vi "GUI_HTU_Steering_Magnets.vi"() -> ()   [LabVIEW 2020]
uses:
  Shared/GUI_Template/GUI_master/tcp_new_data_event.ctl
  Shared/GUI_Template/GUI_master/tcp new data cluster.ctl
panel:
  in  "GUIdevice 18":string="U_VS5V"
  in  "GUIdevice 17":string="U_VS5H"
  in  "Voltage::17":dbl caption="VS5H Voltage" min=-10.0 max=10.0
  in  "Voltage::18":dbl caption="VS5V Voltage" min=-10.0 max=10.0
  in  "Enable_Output::18":enum16{"on", "off"}(ring) caption="Enable VS5V"
  in  "Enable_Output::17":enum16{"on", "off"}(ring) caption="Enable VS5H"
  in  "Current::17":dbl caption="VS5H Current" min=-5.0 max=5.0
  in  "Current::18":dbl caption="VS5V Current" min=-5.0 max=5.0
  in  "Voltage::15":dbl caption="VS4H Voltage" min=-10.0 max=10.0
  in  "Voltage::16":dbl caption="VS4V Voltage" min=-10.0 max=10.0
  in  "Enable_Output::16":enum16{"on", "off"}(ring) caption="Enable VS4V"
  in  "Enable_Output::15":enum16{"on", "off"}(ring) caption="Enable VS4H"
  in  "Current::15":dbl caption="VS4H Current" min=-5.0 max=5.0
  in  "Current::16":dbl caption="VS4V Current" min=-5.0 max=5.0
  in  "Voltage::13":dbl caption="VS3H Voltage" min=-10.0 max=10.0
  in  "Voltage::14":dbl caption="VS3V Voltage" min=-10.0 max=10.0
  in  "Enable_Output::14":enum16{"on", "off"}(ring) caption="Enable VS3V"
  in  "Enable_Output::13":enum16{"on", "off"}(ring) caption="Enable VS3H"
  in  "Current::13":dbl caption="VS3H Current" min=-5.0 max=5.0
  in  "Current::14":dbl caption="VS3V Current" min=-5.0 max=5.0
  in  "Voltage::11":dbl caption="VS2H Voltage" min=-10.0 max=10.0
  in  "Voltage::12":dbl caption="VS2V Voltage" min=-10.0 max=10.0
  in  "Enable_Output::12":enum16{"on", "off"}(ring) caption="Enable VS2V"
  in  "Enable_Output::11":enum16{"on", "off"}(ring) caption="Enable VS2H"
  in  "Current::11":dbl caption="VS2H Current" min=-5.0 max=5.0
  in  "Current::12":dbl caption="VS2V Current" min=-5.0 max=5.0
  in  "GUIdevice 16":string="U_VS4V"
  in  "GUIdevice 15":string="U_VS4H"
  in  "GUIdevice 14":string="U_VS3V"
  in  "GUIdevice 13":string="U_VS3H"
  in  "GUIdevice 12":string="U_VS2V"
  in  "GUIdevice 11":string="U_VS2H"
  in  "GUIdevice 10":string="U_VS1V"
  in  "GUIdevice 9":string="U_VS1H"
  in  "Voltage::9":dbl caption="VS1H Voltage" min=-10.0 max=10.0
  in  "Voltage::10":dbl caption="VS1V Voltage" min=-10.0 max=10.0
  in  "Enable_Output::10":enum16{"on", "off"}(ring) caption="Enable VS1V"
  in  "Enable_Output::9":enum16{"on", "off"}(ring) caption="Enable VS1H"
  in  "Current::9":dbl caption="VS1H Current" min=-5.0 max=5.0
  in  "Current::10":dbl caption="VS1V Current" min=-5.0 max=5.0
  in  "GUIdevice 8":string="U_S4V"
  in  "GUIdevice 7":string="U_S4H"
  in  "Voltage::7":dbl caption="S4H Voltage" min=-10.0 max=10.0
  in  "Voltage::8":dbl caption="S4V Voltage" min=-10.0 max=10.0
  in  "Enable_Output::8":enum16{"on", "off"}(ring) caption="Enable S4V"
  in  "Enable_Output::7":enum16{"on", "off"}(ring) caption="Enable S4H"
  in  "Current::7":dbl caption="S4H Current" min=-5.0 max=5.0
  in  "Current::8":dbl caption="S4V Current" min=-5.0 max=5.0
  in  "GUIdevice 6":string="U_S3V"
  in  "GUIdevice 5":string="U_S3H"
  in  "Voltage::5":dbl caption="S3H Voltage" min=-10.0 max=10.0
  in  "Voltage::6":dbl caption="S3V Voltage" min=-10.0 max=10.0
  in  "Enable_Output::6":enum16{"on", "off"}(ring) caption="Enable S3V"
  in  "Enable_Output::5":enum16{"on", "off"}(ring) caption="Enable S3H"
  in  "Current::5":dbl caption="S3H Current" min=-5.0 max=5.0
  in  "Current::6":dbl caption="S3V Current" min=-5.0 max=5.0
  in  "Voltage::3":dbl caption="S2H Voltage" min=-10.0 max=10.0
  in  "Voltage::4":dbl caption="S2V Voltage" min=-10.0 max=10.0
  in  "Enable_Output::4":enum16{"on", "off"}(ring) caption="Enable S2V"
  in  "Enable_Output::3":enum16{"on", "off"}(ring) caption="Enable S2H"
  in  "Current::3":dbl caption="S2H Current" min=-5.0 max=5.0
  in  "Current::4":dbl caption="S2V Current" min=-5.0 max=5.0
  in  "GUIdevice 4":string="U_S2V"
  in  "GUIdevice 3":string="U_S2H"
  in  "Voltage::1":dbl caption="S1H Voltage" min=-10.0 max=10.0
  in  "Voltage::2":dbl caption="S1V Voltage" min=-10.0 max=10.0
  in  "Enable_Output::2":enum16{"on", "off"}(ring) caption="Enable S1V"
  in  "Enable_Output::1":enum16{"on", "off"}(ring) caption="Enable S1H"
  in  "Current::1":dbl caption="S1H Current" min=-5.0 max=5.0
  in  "Current::2":dbl caption="S1V Current" min=-5.0 max=5.0
  out "error IO 2":errorcluster
  out "tcp data event":T1
  in  "UDP error message":string
  in  "GUIdevice 2":string="U_S1V"
  in  "GUIdevice 1":string="U_S1H"
  in  "stop":bool
  # "Energy"
  # "HTU Steering Magnets"
  # "S1H"
  # "S1V"
  # "S2H"
  # "S2V"
  # "S3H"
  # "S3V"
  # "S4H"
  # "S4V"
  # "Enable output"
  # "Current"
  # "Voltage"
  # "VS1H"
  # "VS1V"
  # "VS2H"
  # "VS2V"
  # "VS3H"
  # "VS3V"
  # "VS4H"
  # "VS4V"
  # "VS5H"
  # "VS5V"
  # "Enable output"
  # "Current"
  # "Voltage"
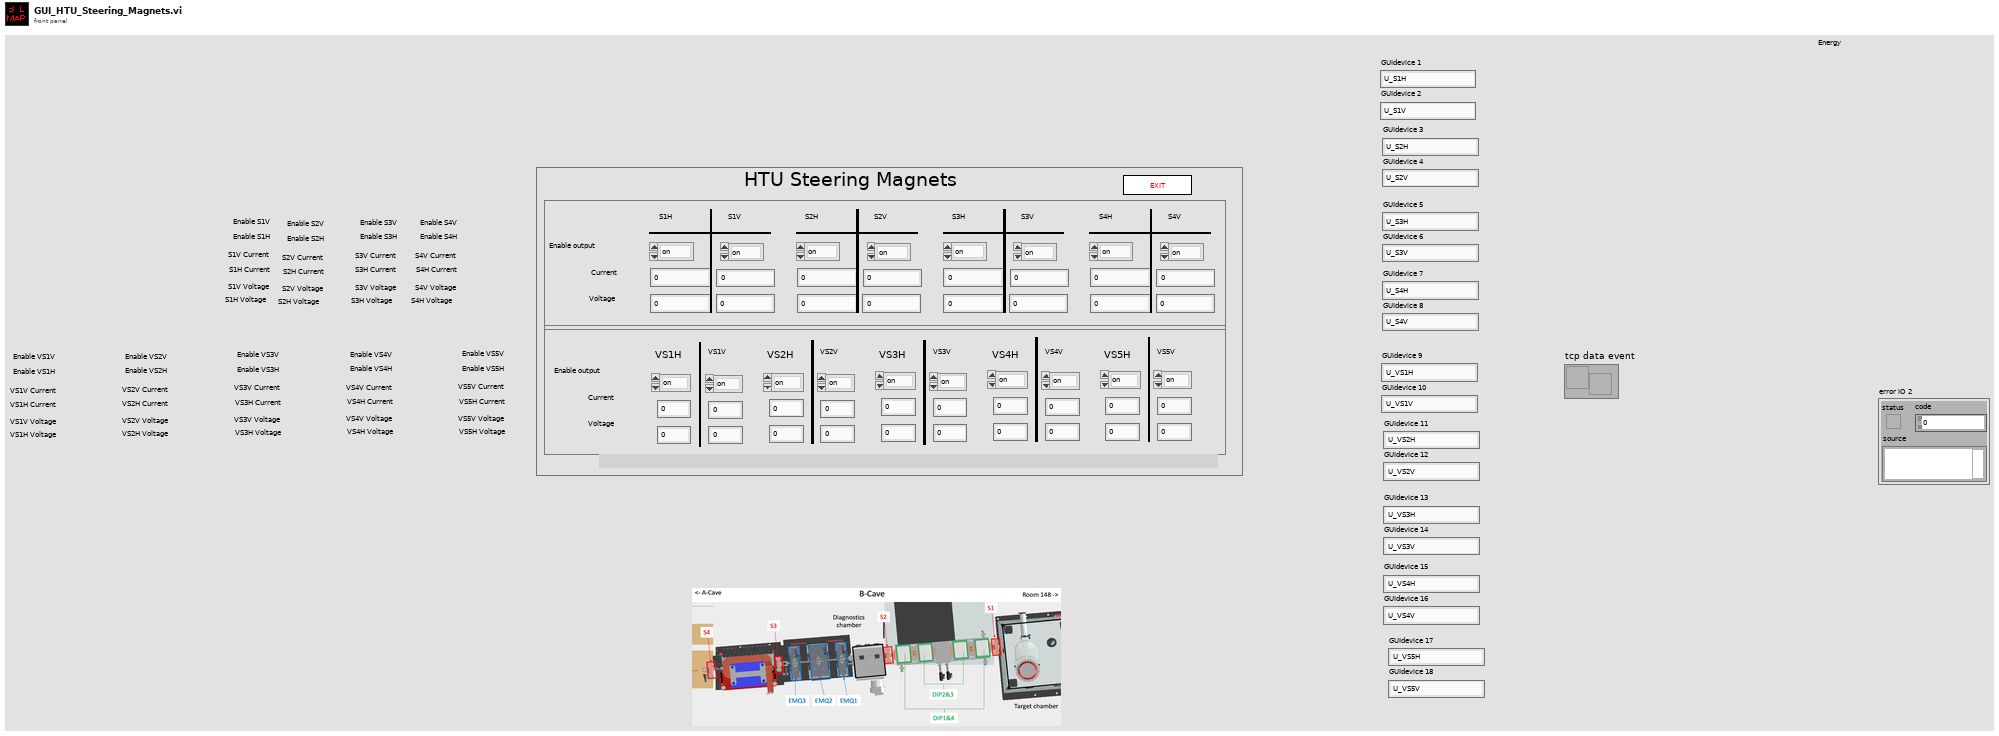
[diagram p1: front panel]
types:
  T1 = typedef "tcp_new_data_event.ctl" = refnum<user-event>
  T2 = typedef "tcp new data cluster.ctl" = cluster{"EventEnum":enum16{"new data", "connection status update"}, "Device name":string}
  T3 = enum32{"invalid app kind", "Development System", "Run Time System", "Student Edition", "Embedded LabVIEW", "Evaluation", "Custom"}
  T4 = enum32{"Invalid", "Standard", "Closed", "Hidden", "Minimized", "Maximized"}
  T5 = cluster{"Core":cluster{"Current VI Reference":refnum<vi>, "Close Panel on Exit?":bool}}
  T6 = cluster{"Current VI Reference":refnum<vi>, "Close Panel on Exit?":bool}
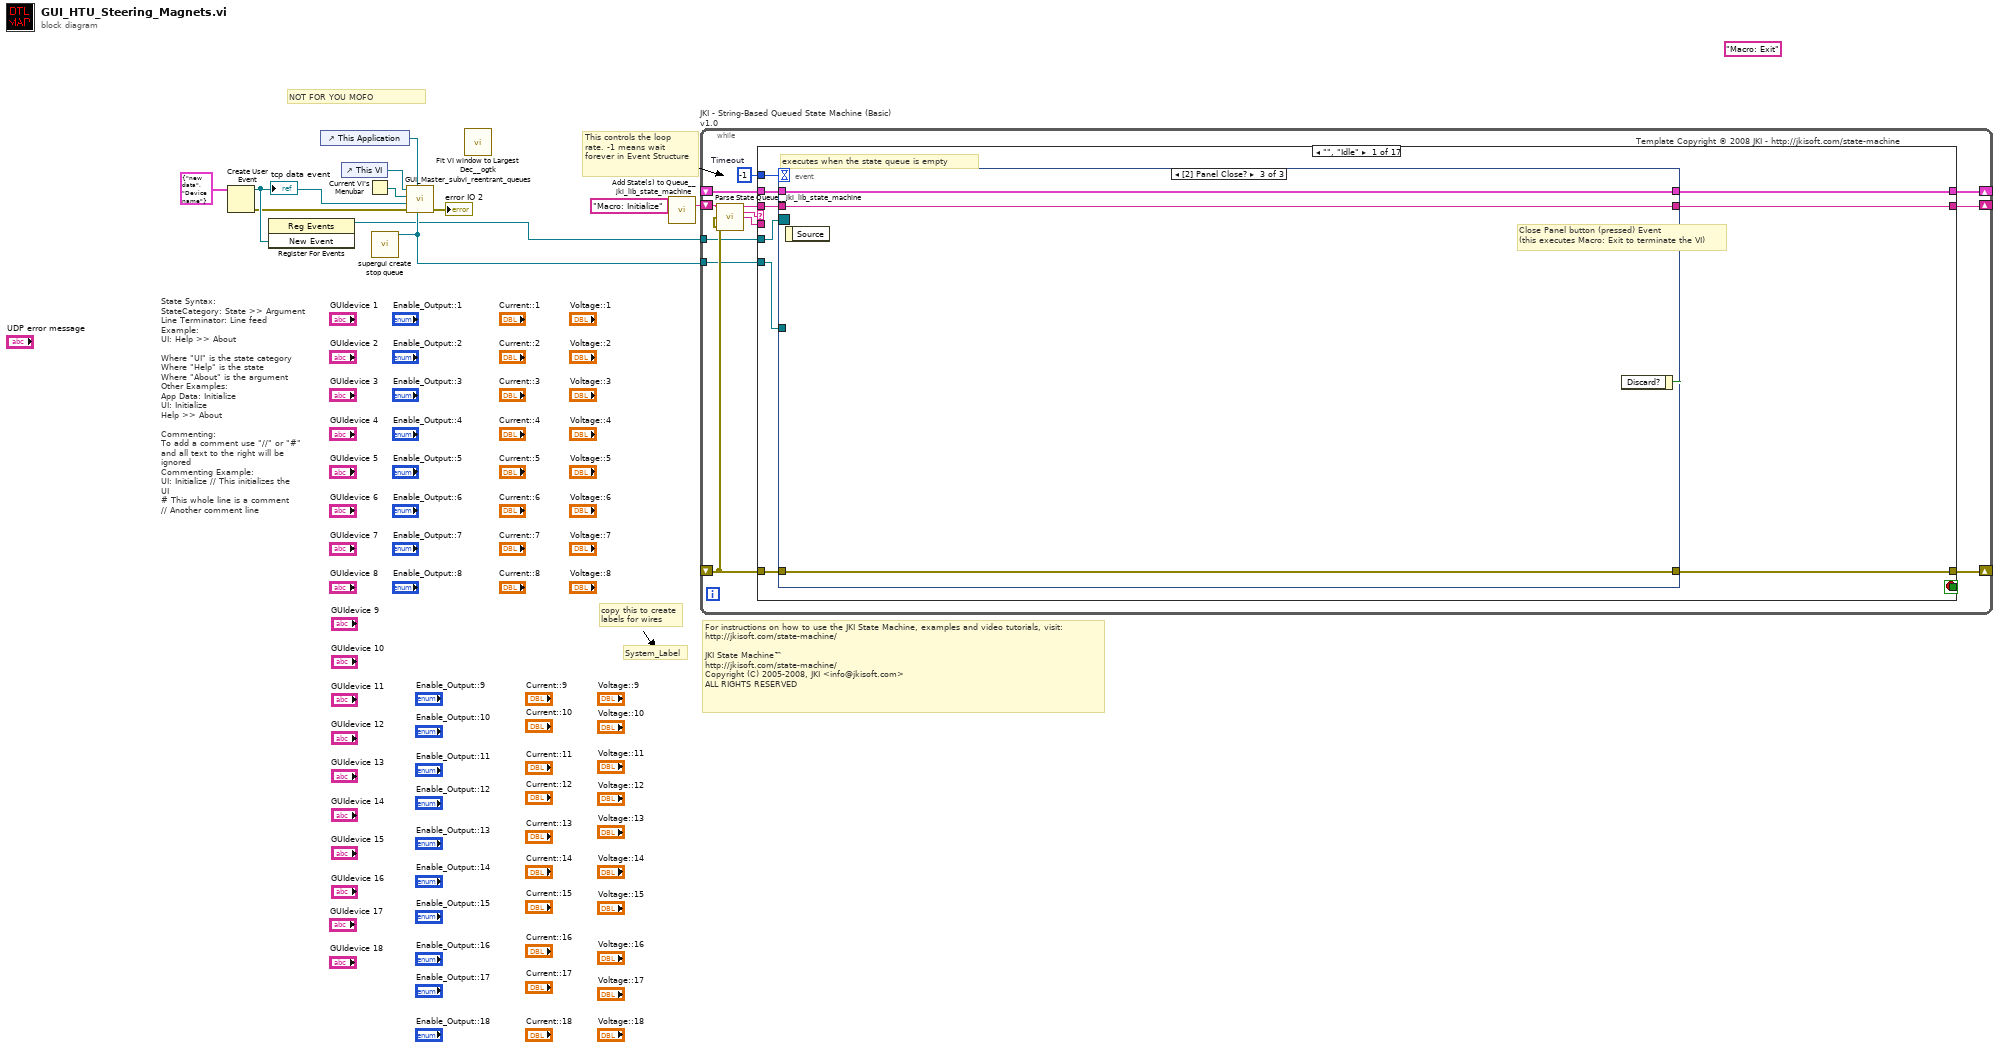
[diagram p0: block diagram]
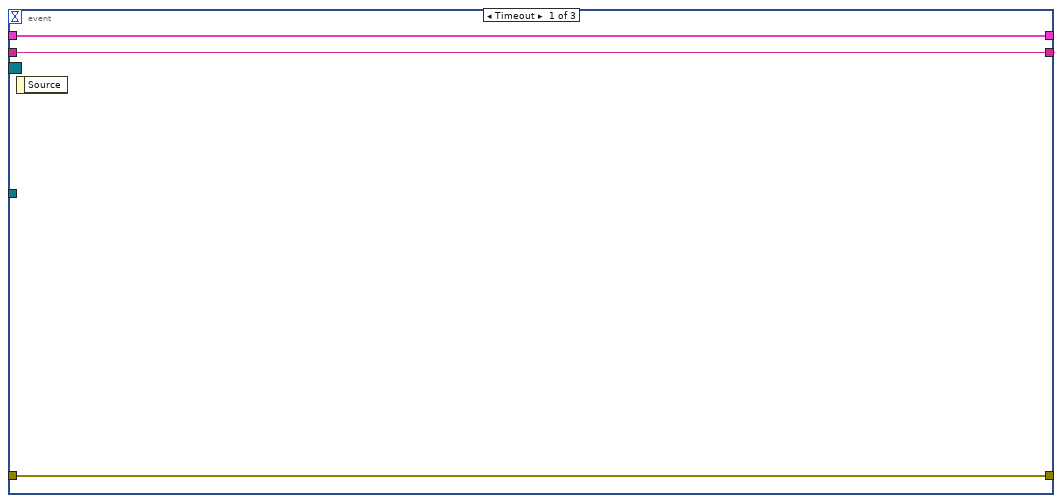
[diagram p2: hidden frame]
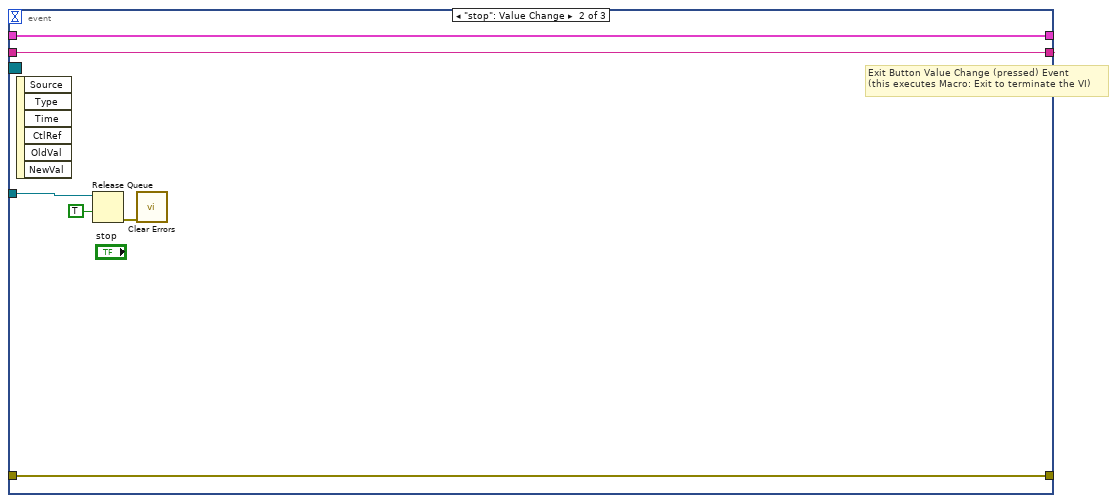
[diagram p3: hidden frame]
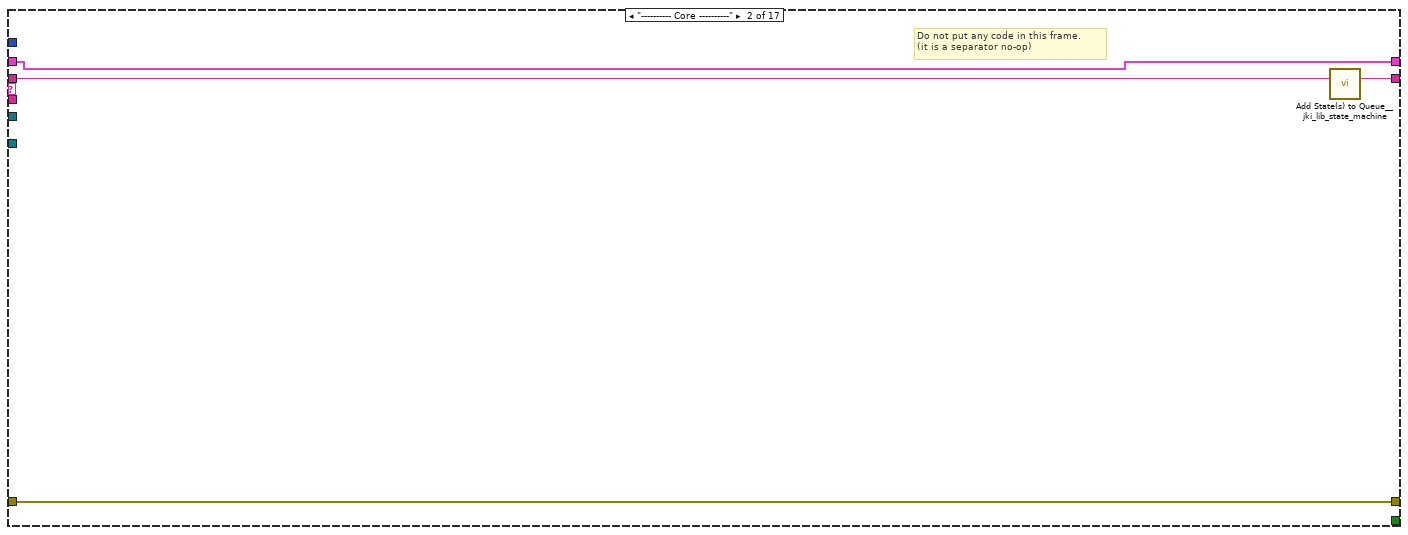
[diagram p4: hidden frame]
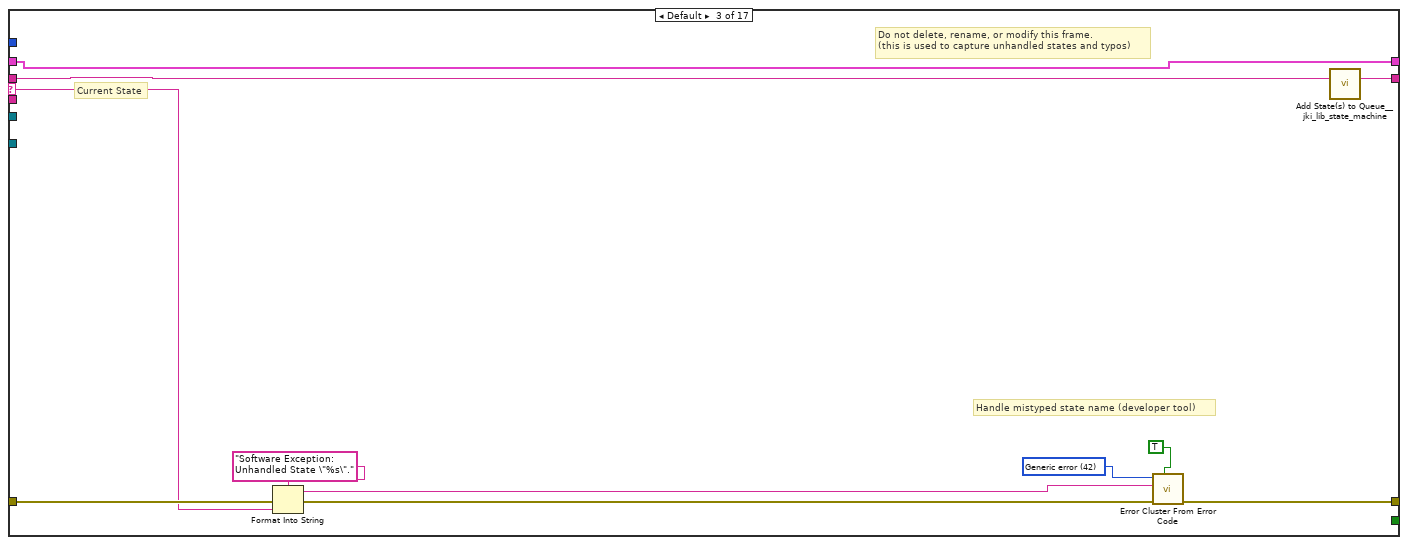
[diagram p5: hidden frame]
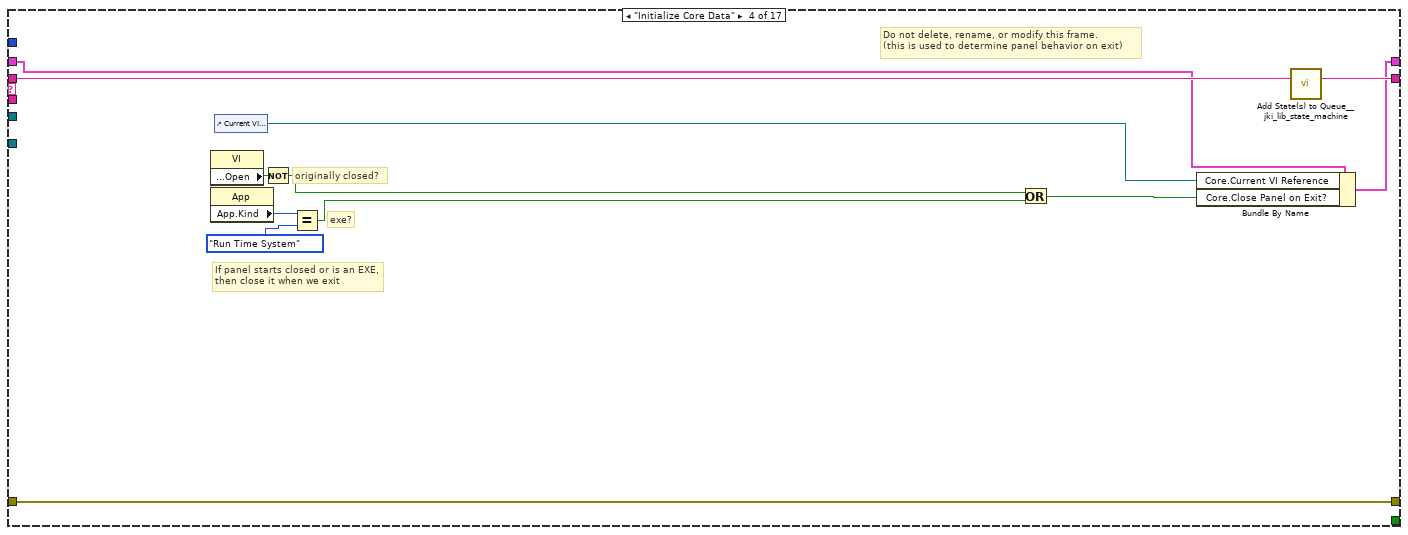
[diagram p6: hidden frame]
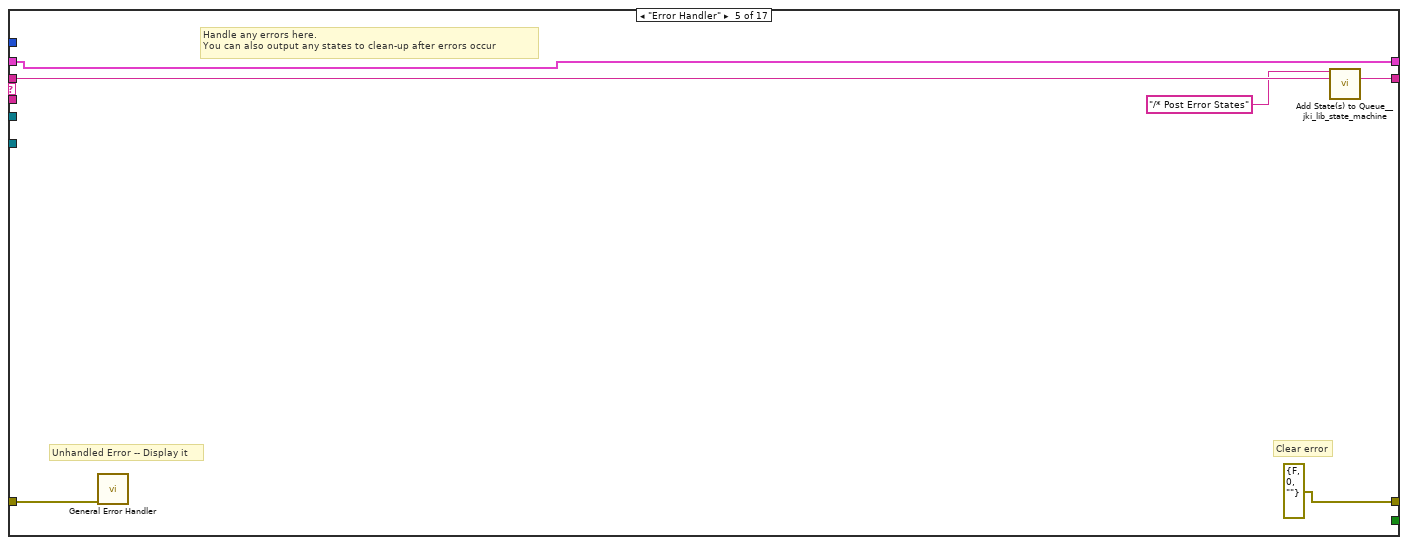
[diagram p7: hidden frame]
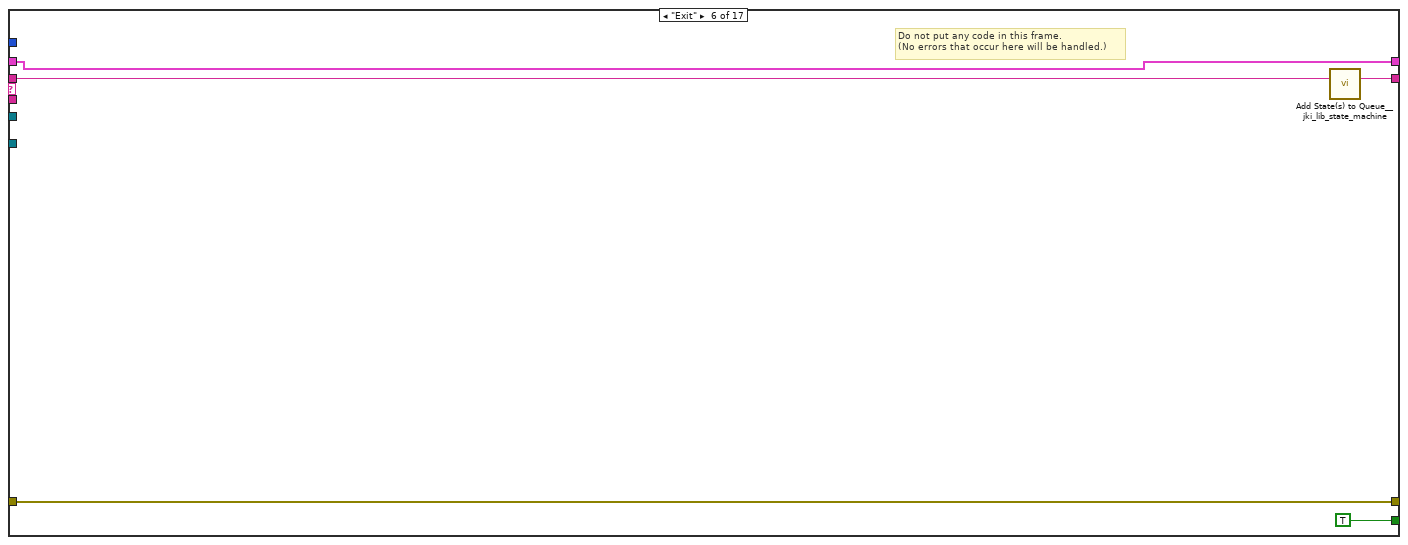
[diagram p8: hidden frame]
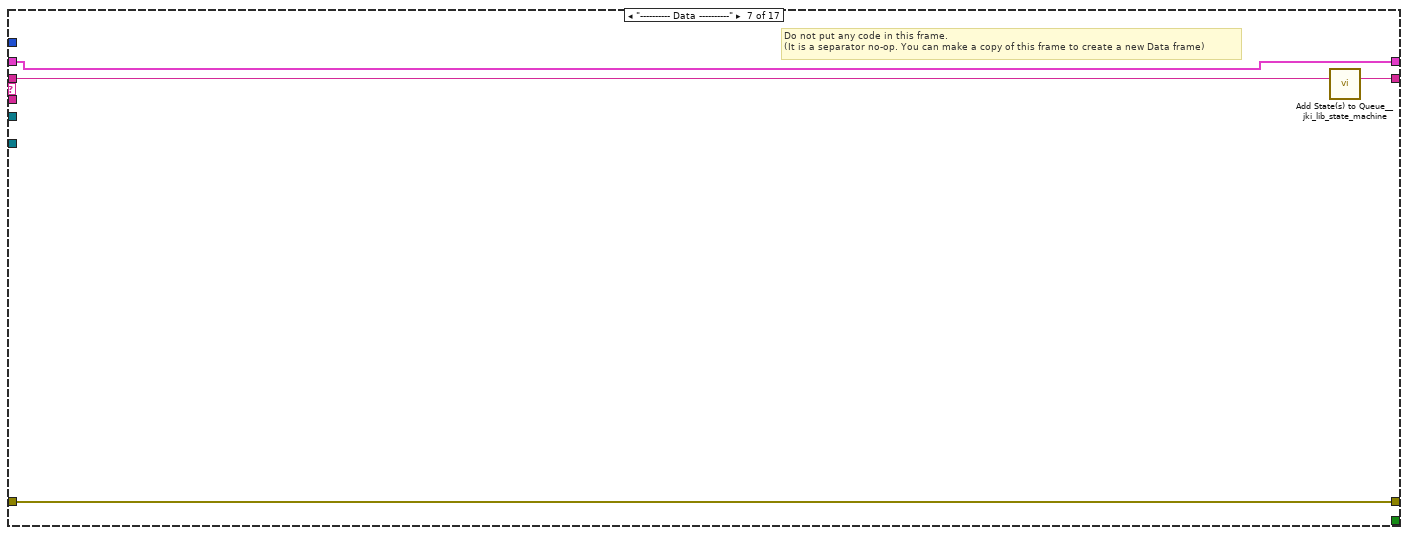
[diagram p9: hidden frame]
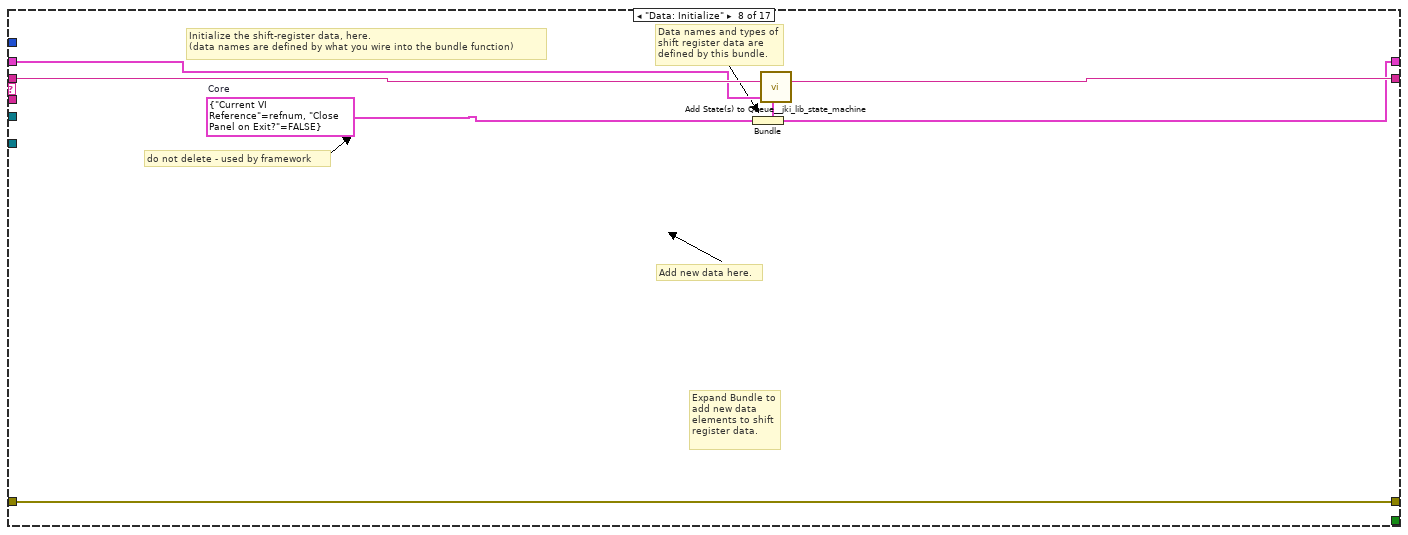
[diagram p10: hidden frame]
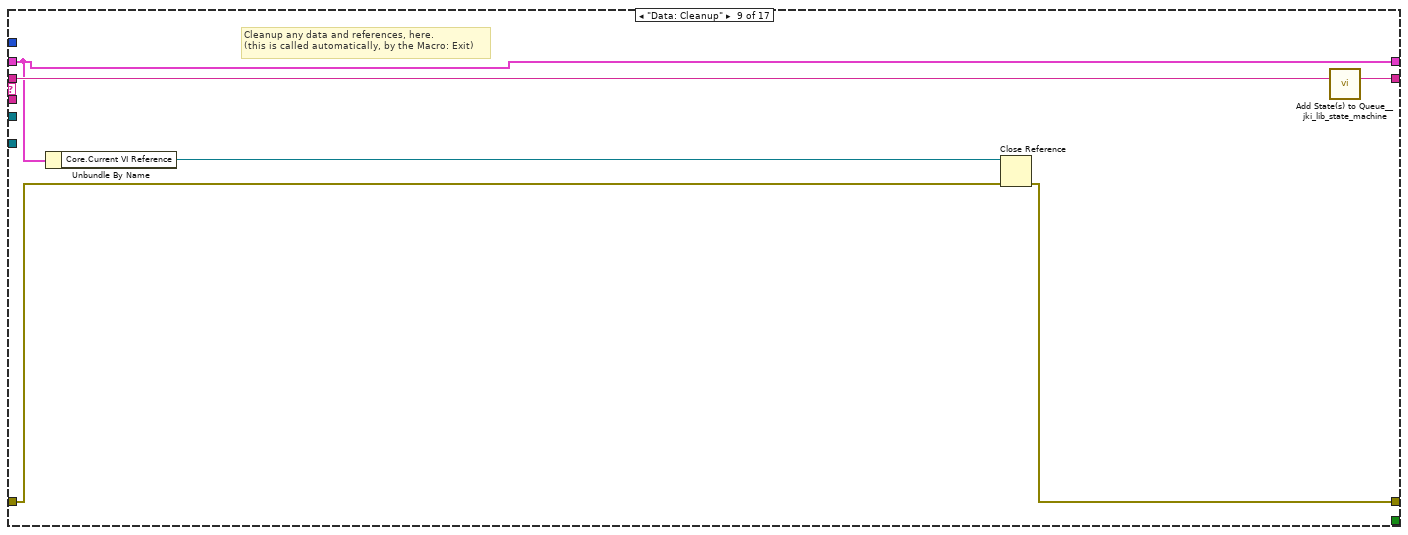
[diagram p11: hidden frame]
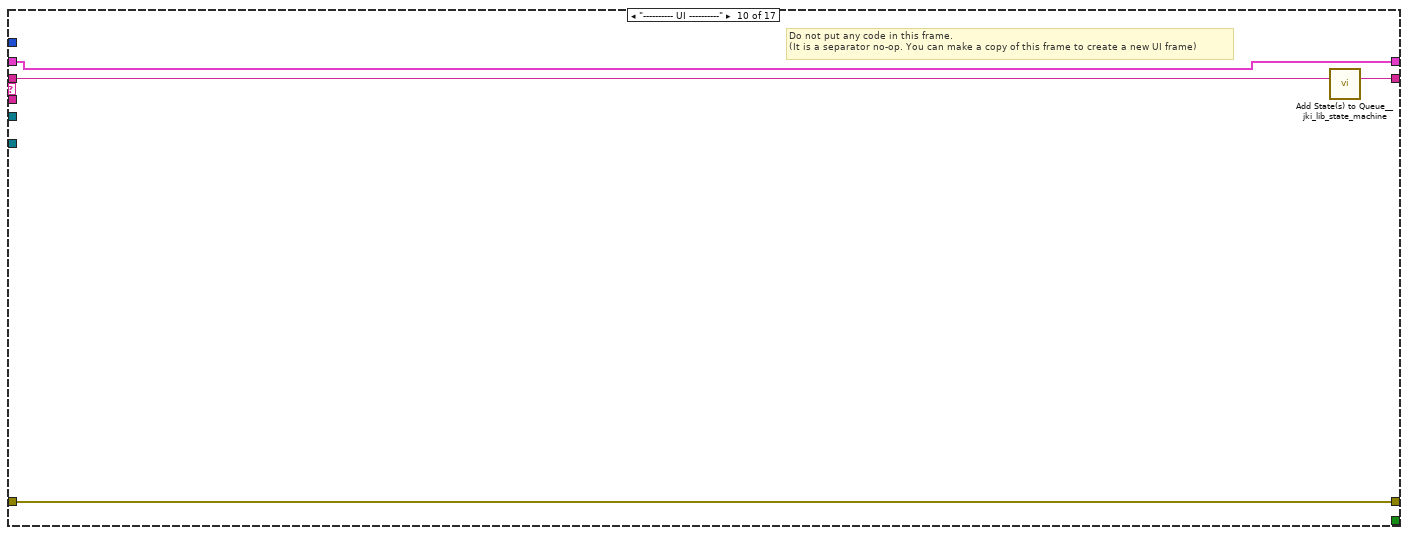
[diagram p12: hidden frame]
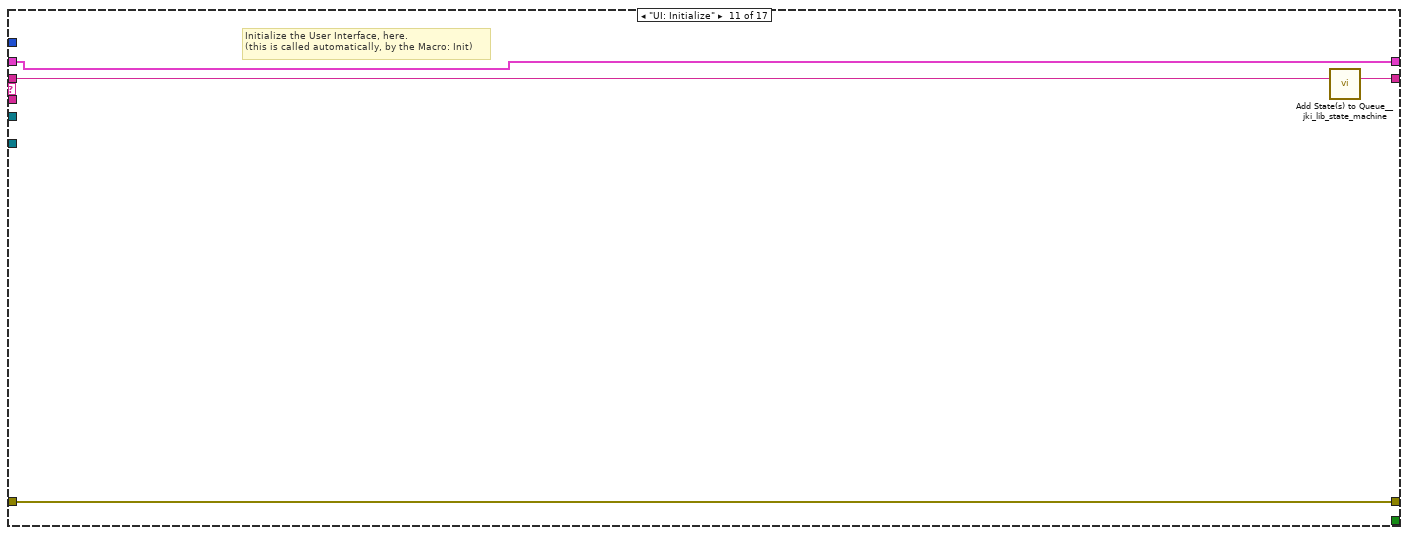
[diagram p13: hidden frame]
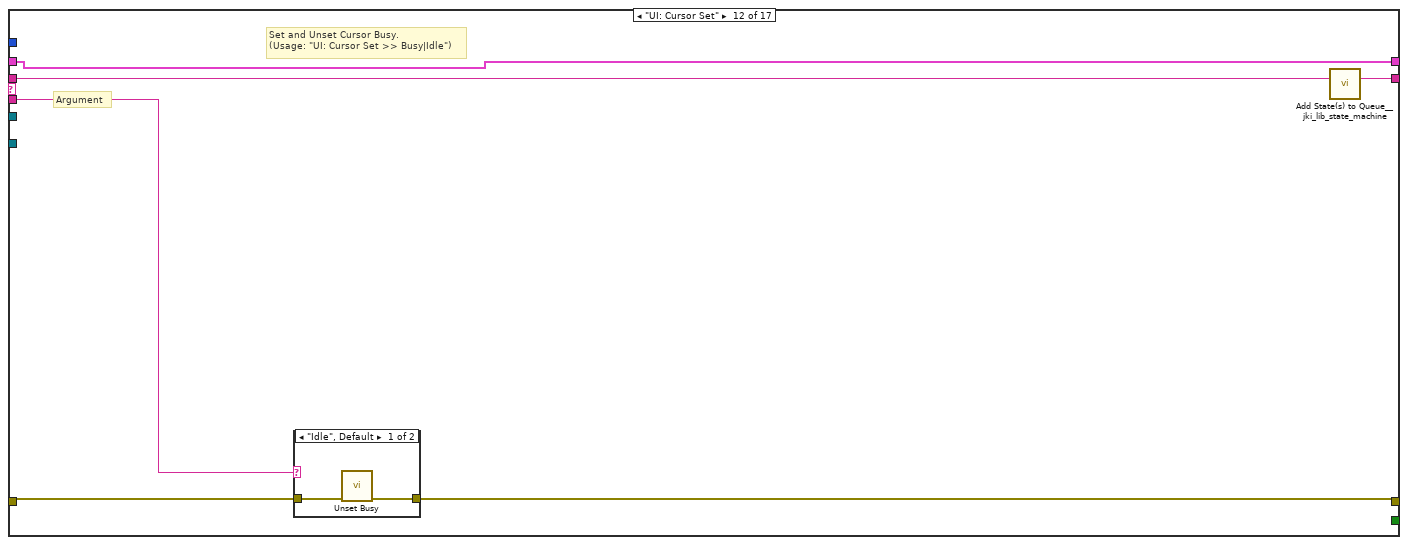
[diagram p14: hidden frame]
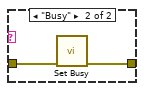
[diagram p15: hidden frame]
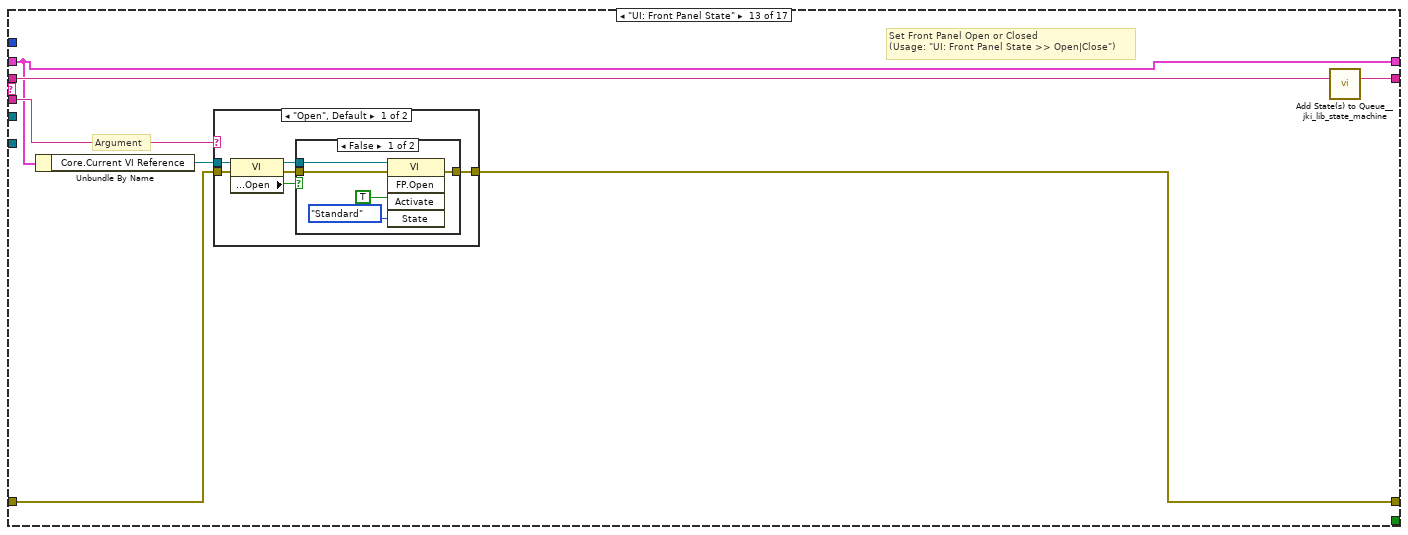
[diagram p16: hidden frame]
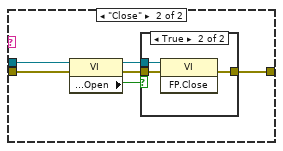
[diagram p18: hidden frame]
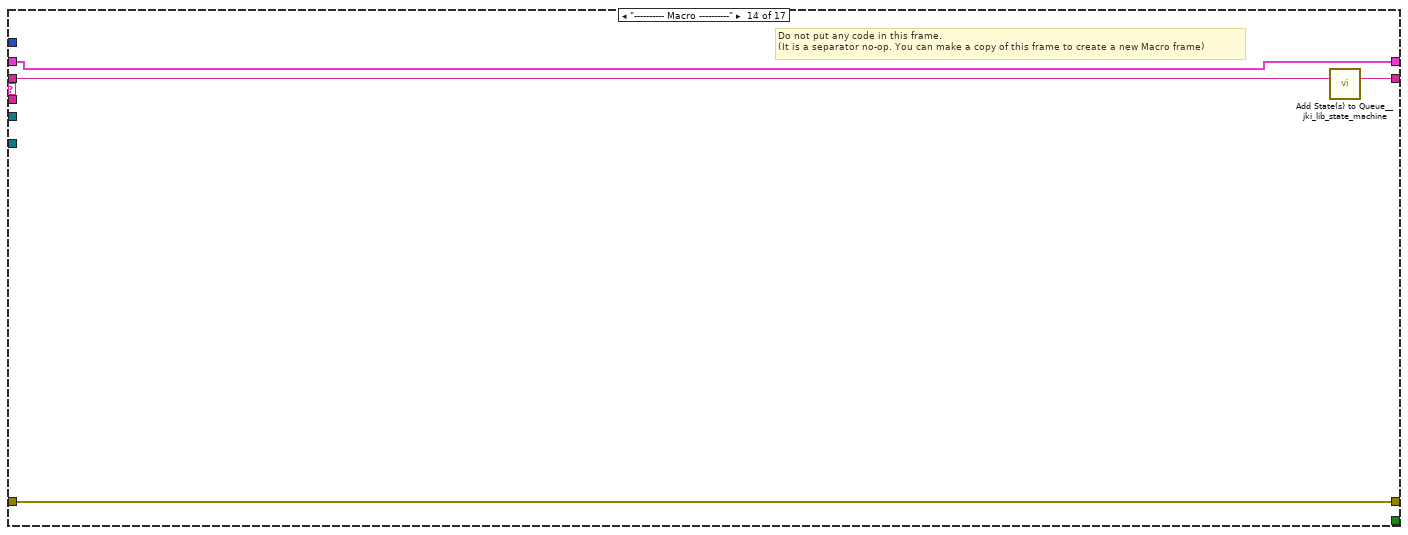
[diagram p20: hidden frame]
diagram:
  (unwired) "Macro: Exit"
  # "For instructions on how to use the JKI State Machine, examples and video tutorials, visit:\nhttp://jkisoft.com/state-machine/\n\nJKI State Machine™\nhttp://jkisoft.com/state-machine/\nCopyright (C) 2005-2008, JKI <info@jkisoft.com>\nALL RIGHTS RESERVED"
  # "State Syntax:\nStateCategory: State >> Argument\nLine Terminator: Line feed\nExample:\nUI: Help >> About\n\nWhere \"UI\" is the state category\nWhere \"Help\" is the state\nWhere \"About\" is the argument\nOther Examples:\nApp Data: Initialize\nUI: Initialize\nHelp >> About\n\nCommenting:\nTo add a comment use \"//\" or \"#\" and all text to the right will be ignored\nCommenting Example:\nUI: Initialize // This initializes the UI\n# This whole line is a comment\n// Another comment line"
  # "copy this to create labels for wires"
  # "This controls the loop rate. -1 means wait forever in Event Structure"
  # "System_Label"
  # "NOT FOR YOU MOFO"
  n1 = Create User Event(user event datatype=T2 {"EventEnum"=enum."new data", "Device name"="Device name"} ("New Event")) -> (user event=w10:refnum<user-event>, error out=w9:errorcluster)  [unwired: 1 in]
  "tcp data event" <- w10
  n2 = register-events(w10) -> (reference out=w1:refnum<event-registration>)  [unwired: 2 in, 1 out]
  n3 = control-ref of="This Application"() -> (w11:refnum<vi>)
  n4 = control-ref of="This VI"() -> (w5:refnum<vi>)
  n5 = Current VI's Menubar() -> (w7:refnum<k9>)
  n6 = call "supergui create stop queue.vi"() -> ("STOP Queue out"=w2:refnum<queue>)  [unwired: 11 in]
  n7 = call "GUI_Master_subvi_reentrant_queues.vi"("STOP Queue in"=w2, "This Application"=w11, "error in (no error)"=w9, "tcp data event"=w10, "Caller menu reference"=w7, "Caller VI ref"=w5) -> ("error out"=→"error IO 2":errorcluster)  [unwired: 5 in]
  n8 = call <userlib>:"Fit VI window to Largest Dec__ogtk.vi"() -> ()  [unwired: 6 in, 2 out]
  n9 = call <vilib>:"Add State(s) to Queue__jki_lib_state_machine.vi"("State(s) in (\"\")"="Macro: Initialize") -> ("States Out"=w3:string)  [unwired: 14 in]
  n10 = while "JKI - String-Based Queued State Machine (Basic) v1.0" {
    shift-right: [w17] -> _
    shift-left: _ -> [w16]
    shift-right: [w20] -> _
    shift-left: _ -> [w14]
    shift-right: [w19] -> _
    shift-left: w3 -> [w21]
    tunnel: w1 -> [w13]
    tunnel: w2 -> [w12]
    stop <- w18 stop-if-true
    w15 = -1  # Timeout
    # "Template Copyright © 2008 JKI - http://jkisoft.com/state-machine"
    n11 = call <vilib>:"Parse State Queue__jki_lib_state_machine.vi"("State Queue"=w21, "Error In (no error)"=w14) -> ("Remaining States"=w23:string, "Current State"=w24:string, "Arguments"=w22:string)  [unwired: 11 in]
    n12 = case shown="\"\", \"Idle\"" w24 {
      selector: w24 -> [_ _ w56 _ _ _ _ _ _ _ _ _ _ _ _ _ _]
      tunnel: w23 -> [w33 w55 w60 w78 w84 w89 w93 w99 w105 w109 w113 w119 w130 w156 w161 w171 w175]
      tunnel: w22 -> [_ _ _ _ _ _ _ _ _ _ _ w114 w125 _ _ _ _]
      tunnel: w16 -> [w31 w52 w58 w68 w81 w87 w90 w95 w100 w106 w111 w117 w124 w153 w158 w162 w172]
      tunnel: [w30 w53 w62 w76 errorcluster {"status"=FALSE, "code"=0, "source"=""} ("error out") w86 w91 w97 w102 w107 w110 w115 w127 w154 w159 w169 w173] -> w20
      tunnel: w14 -> [w29 w53 w61 w76 w80 w86 w91 w97 w103 w107 w110 w116 w128 w154 w159 w169 w173]
      tunnel: [w32 w54 w59 w77 w83 w88 w92 w98 w104 w108 w112 w118 w129 w155 w160 w170 w174] -> w19
      tunnel: [_ _ _ _ _ TRUE _ _ _ _ _ _ _ _ _ _ _] -> w18
      tunnel: [w25 w52 w58 w67 w81 w87 w90 w94 w100 w106 w111 w117 w124 w153 w158 w162 w172] -> w17
      tunnel: w15 -> [w28 _ _ _ _ _ _ _ _ _ _ _ _ _ _ _ _]
      tunnel: w13 -> [w27 _ _ _ _ _ _ _ _ _ _ _ _ _ _ _ _]
      tunnel: w12 -> [w26 _ _ _ _ _ _ _ _ _ _ _ _ _ _ _ _]
      frame "", "Idle" {
        # "executes when the state queue is empty"
        n13 = event shown="[2] Panel Close?" {
          selector: w27 -> [_ _ _]
          dyn-events: _ -> [_ _ _]
          timeout: w28 -> [_ _ _]
          tunnel: w33 -> [w37 w45 w51]
          tunnel: [w36 w44 w50] -> w32
          tunnel: w31 -> [w34 w42 w48]
          tunnel: [w35 w43 w49] -> w30
          tunnel: w29 -> [w35 w43 w49]
          tunnel: [w34 w42 w48] -> w25
          tunnel: w26 -> [_ w39 _]
          event Timeout {
            n14 = event-data() -> ()  [unwired: 1 in, 1 out]
            n15 = call <vilib>:"Add State(s) to Queue__jki_lib_state_machine.vi"("State(s) in (\"\")"=w37) -> ("States Out"=w36:string)  [unwired: 14 in]
          }
          event "stop": Value Change {
            # "Exit Button Value Change (pressed) Event\n(this executes Macro: Exit to terminate the VI)"
            n16 = event-data() -> ()  [unwired: 1 in, 6 out]
            n17 = Release Queue(queue=w39, force destroy? (F)=TRUE) -> (error out=w40:errorcluster)  [unwired: 1 in, 2 out]
            n18 = call <vilib>:"Clear Errors.vi"("error in (no error)"=w40) -> ()  [unwired: 5 in, 2 out]
            n19 = call <vilib>:"Add State(s) to Queue__jki_lib_state_machine.vi"("State(s) in Front (\"\")"="Macro: Exit", "State(s) in (\"\")"=w45) -> ("States Out"=w44:string)  [unwired: 13 in]
          }
          event Panel Close? {
            # "Discard the event because we'll close the front panel ourselves in Macro: Exit"
            # "Close Panel button (pressed) Event\n(this executes Macro: Exit to terminate the VI)"
            n20 = event-data() -> ()  [unwired: 1 in, 1 out]
            n21 = event-data("Discard?"=TRUE) -> ()  [unwired: 1 in, 1 out]
            n22 = call <vilib>:"Add State(s) to Queue__jki_lib_state_machine.vi"("State(s) in Front (\"\")"="Macro: Exit", "State(s) in (\"\")"=w51) -> ("States Out"=w50:string)  [unwired: 13 in]
          }
        }
      }
      frame "---------- Core ----------" {
        # "Do not put any code in this frame.\n(it is a separator no-op)"
        n23 = call <vilib>:"Add State(s) to Queue__jki_lib_state_machine.vi"("State(s) in (\"\")"=w55) -> ("States Out"=w54:string)  [unwired: 14 in]
      }
      frame Default {
        w65 = 42 items=["No error", "Argument error", "Memory is full", "Out of zone", "End of file", "File already open", "Generic file I/O error", "File not found", "File permission error", "Disk is full", "Duplicate path", "Too many files open", "System feature not enabled", "Resource file not found", "Cannot add resource", "Resource not found", "Image not found", "Image memory error", "Pen does not exist", "Config type invalid", "Config token not found", "Config parse error", "Config memory error", "Bad external code format", "Bad external code offset", "External code not present", "Null window", "Destroy window error", "Null menu", "Print aborted", "Bad print record", "Print driver error", "Windows error during printing", "Memory error during printing", "Print dialog error", "Generic print error", "Invalid device refnum", "Device not found", "Device parameter error", "Device unit error", "Cannot open device", "Device call aborted", "Generic error", "Cancelled by user", "Object ID too low", "Object ID too high", "Object not in heap", "Unknown heap", "Unknown object (invalid DefProc)", "Unknown object (DefProc not in table)", "Message out of range", "Invalid (null) method", "Unknown message", "Manager call not supported", "Bad address", "Network operation in progress", "Network operation timed out", "Connection is busy", "Network attribute not supported", "Network error", "Address in use", "System out of memory", "Connection aborted", "Connection refused", "Not connected", "Already connected", "Connection closed", "Initialization error (interapplication manager)", "Bad occurrence", "Wait on unbound occurrence handler", "Occurrence queue overflow", "Datalog type conflict", "Unused", "Unrecognized type (interapplication manager)", "Memory corrupt", "Failed to make temporary DLL", "Old CIN version", "Drag socket not found", "Failed to load drop-object", "Failed to register OLE object", "Failed to release OLE object", "Format specifier type mismatch", "Unknown format specifier", "Too few format specifiers", "Too many format specifiers", "Scan failed", "Newer CIN version", "Error converting to variant", "Runtime menu error", "Password tampered", "Variant attribute not found", "Incompatible variant data type", "Event data is not available", "Event Store is not present", "Occurrence is not found", "Event Queue is not created", "Event info is not available", "Refnum passed is NULL", "Error retrieving Class GUID", "Error retrieving CoClass GUID", "Error retrieving TypeLib GUID.", "Bad built application magic bytes.", "Specific driver is different from the specific driver associated with the Logical Name.", "There is no session opened to the class driver.", "Max Error", "MAX - Error with config objects", "MAX - Error loading configuration", "MAX - Group not supported"]
        # "Current State"
        # "Do not delete, rename, or modify this frame.\n(this is used to capture unhandled states and typos)"
        # "Handle mistyped state name (developer tool)"
        n24 = Format Into String(format string="Software Exception: Unhandled State \"%s\"." ("message"), error in=w61, w56) -> (resulting string=w64:string, error out=w63:errorcluster)  [unwired: 1 in]
        n25 = call <vilib>:"Error Cluster From Error Code.vi"("show call chain? (False)"=TRUE, "error in (no error)"=w63, "error message (\"\")"=w64, "error code (0)"=w65) -> ("error out"=w62:errorcluster)  [unwired: 5 in]
        n26 = call <vilib>:"Add State(s) to Queue__jki_lib_state_machine.vi"("State(s) in (\"\")"=w60) -> ("States Out"=w59:string)  [unwired: 14 in]
      }
      frame "Initialize Core Data" {
        # "Do not delete, rename, or modify this frame.\n(this is used to determine panel behavior on exit)"
        # "originally closed?"
        # "exe?"
        # "If panel starts closed or is an EXE, then close it when we exit"
        n27 = property class="VI"() -> ("Front Panel.Open"=w75:bool)  [unwired: 2 in, 2 out]
        n28 = property class="App"() -> ("App.Kind"=w74:T3)  [unwired: 2 in, 2 out]
        n29 = control-ref of="Current VI Reference"() -> (w69:refnum<vi>)
        n30 = Not(x=w75) -> (.not. x?=w72:bool)
        n31 = Equal?(x=w74, y=T3."Run Time System" ("Application:Kind")) -> (x = y?=w71:bool)
        n32 = Or(x=w72, y=w71) -> (x .or. y?=w70:bool)
        n33 = Bundle By Name(cluster=w68, "Core.Current VI Reference"=w69, "Core.Close Panel on Exit?"=w70) -> (w67:T5)
        n34 = call <vilib>:"Add State(s) to Queue__jki_lib_state_machine.vi"("State(s) in (\"\")"=w78) -> ("States Out"=w77:string)  [unwired: 14 in]
      }
      frame "Error Handler" {
        # "Unhandled Error -- Display it"
        # "Handle any errors here.\nYou can also output any states to clean-up after errors occur"
        # "Clear error"
        n35 = call <vilib>:"General Error Handler.vi"("error in (no error)"=w80) -> ()  [unwired: 10 in, 5 out]
        n36 = call <vilib>:"Add State(s) to Queue__jki_lib_state_machine.vi"("State(s) in Front (\"\")"="/* Post Error States", "State(s) in (\"\")"=w84) -> ("States Out"=w83:string)  [unwired: 13 in]
      }
      frame "Exit" {
        # "Do not put any code in this frame.\n(No errors that occur here will be handled.)"
        n37 = call <vilib>:"Add State(s) to Queue__jki_lib_state_machine.vi"("State(s) in (\"\")"=w89) -> ("States Out"=w88:string)  [unwired: 14 in]
      }
      frame "---------- Data ----------" {
        # "Do not put any code in this frame.\n(It is a separator no-op. You can make a copy of this frame to create a new Data frame)"
        n38 = call <vilib>:"Add State(s) to Queue__jki_lib_state_machine.vi"("State(s) in (\"\")"=w93) -> ("States Out"=w92:string)  [unwired: 14 in]
      }
      frame "Data: Initialize" {
        w96 = T6 {"Current VI Reference"=refnum, "Close Panel on Exit?"=FALSE}  # Core
        # "do not delete - used by framework"
        # "Expand Bundle to add new data elements to shift register data."
        # "Add new data here."
        # "Data names and types of shift register data are defined by this bundle."
        # "Initialize the shift-register data, here.\n(data names are defined by what you wire into the bundle function)"
        n39 = Bundle(cluster=w95, "Core"=w96) -> (w94:T5)
        n40 = call <vilib>:"Add State(s) to Queue__jki_lib_state_machine.vi"("State(s) in (\"\")"=w99) -> ("States Out"=w98:string)  [unwired: 14 in]
      }
      frame "Data: Cleanup" {
        # "Cleanup any data and references, here.\n(this is called automatically, by the Macro: Exit)"
        n41 = Unbundle By Name(w100) -> ("Core.Current VI Reference"=w101:refnum<vi>)
        n42 = Close Reference(reference=w101, error in (no error)=w103) -> (error out=w102:errorcluster)
        n43 = call <vilib>:"Add State(s) to Queue__jki_lib_state_machine.vi"("State(s) in (\"\")"=w105) -> ("States Out"=w104:string)  [unwired: 14 in]
      }
      frame "---------- UI ----------" {
        # "Do not put any code in this frame.\n(It is a separator no-op. You can make a copy of this frame to create a new UI frame)"
        n44 = call <vilib>:"Add State(s) to Queue__jki_lib_state_machine.vi"("State(s) in (\"\")"=w109) -> ("States Out"=w108:string)  [unwired: 14 in]
      }
      frame "UI: Initialize" {
        # "Initialize the User Interface, here.\n(this is called automatically, by the Macro: Init)"
        n45 = call <vilib>:"Add State(s) to Queue__jki_lib_state_machine.vi"("State(s) in (\"\")"=w113) -> ("States Out"=w112:string)  [unwired: 14 in]
      }
      frame "UI: Cursor Set" {
        # "Argument"
        # "Set and Unset Cursor Busy.\n(Usage: \"UI: Cursor Set >> Busy|Idle\")"
        n46 = case shown="\"Idle\", Default" w114 {
          tunnel: w116 -> [w121 w123]
          tunnel: [w120 w122] -> w115
          frame "Idle", Default {
            n47 = call <vilib>:"Unset Busy.vi"("error in (no error)"=w121) -> ("error out"=w120:errorcluster)  [unwired: 10 in]
          }
          frame "Busy" {
            n48 = call <vilib>:"Set Busy.vi"("error in (no error)"=w123) -> ("error out"=w122:errorcluster)  [unwired: 9 in, 1 out]
          }
        }
        n49 = call <vilib>:"Add State(s) to Queue__jki_lib_state_machine.vi"("State(s) in (\"\")"=w119) -> ("States Out"=w118:string)  [unwired: 14 in]
      }
      frame "UI: Front Panel State" {
        # "Argument"
        # "Set Front Panel Open or Closed\n(Usage: \"UI: Front Panel State >> Open|Close\")"
        n50 = Unbundle By Name(w124) -> ("Core.Current VI Reference"=w126:refnum<vi>)
        n51 = case shown="\"Open\", Default" w125 {
          tunnel: w128 -> [w135 w147]
          tunnel: [w136 w148] -> w127
          tunnel: w126 -> [w131 w143]
          frame "Open", Default {
            n52 = property class="VI"(reference=w131, error in=w135) -> (reference out=w133:refnum<vi>, error out=w134:errorcluster, "Front Panel.Open"=w132:bool)
            n53 = case shown="False" w132 {
              tunnel: [w139 w142] -> w136
              tunnel: w134 -> [w138 w142]
              tunnel: w133 -> [w137 _]
              frame False {
                n54 = invoke class="VI" method="FP.Open"(reference=w137, error in=w138, "Activate"=TRUE, "State"=T4."Standard") -> (error out=w139:errorcluster)  [unwired: 1 in, 4 out]
              }
              frame True {
              }
            }
          }
          frame "Close" {
            n55 = property class="VI"(reference=w143, error in=w147) -> (reference out=w145:refnum<vi>, error out=w146:errorcluster, "Front Panel.Open"=w144:bool)
            n56 = case shown="True" w144 {
              tunnel: [w149 w152] -> w148
              tunnel: w146 -> [w149 w151]
              tunnel: w145 -> [_ w150]
              frame False {
              }
              frame True {
                n57 = invoke class="VI" method="FP.Close"(reference=w150, error in=w151) -> (error out=w152:errorcluster)  [unwired: 1 in, 2 out]
              }
            }
          }
        }
        n58 = call <vilib>:"Add State(s) to Queue__jki_lib_state_machine.vi"("State(s) in (\"\")"=w130) -> ("States Out"=w129:string)  [unwired: 14 in]
      }
      frame "---------- Macro ----------" {
        # "Do not put any code in this frame.\n(It is a separator no-op. You can make a copy of this frame to create a new Macro frame)"
        n59 = call <vilib>:"Add State(s) to Queue__jki_lib_state_machine.vi"("State(s) in (\"\")"=w156) -> ("States Out"=w155:string)  [unwired: 14 in]
      }
      frame "Macro: Initialize" {
        w157 = "Data: Initialize\nInitialize Core Data\nUI: Initialize\nUI: Front Panel State >> Open"  # Data: Initialize Initialize Core Data UI: Initialize UI: Front Panel State >> Open
        # "Initialization Macro\n(This is called once, when the VI starts)"
        n60 = call <vilib>:"Add State(s) to Queue__jki_lib_state_machine.vi"("State(s) in Front (\"\")"=w157, "State(s) in (\"\")"=w161) -> ("States Out"=w160:string)  [unwired: 13 in]
      }
      frame "Macro: Exit" {
        # "Exit Macro\n(This is called once, when the VI exits)"
        n61 = Unbundle By Name(w162) -> ("Core.Close Panel on Exit?"=w163:bool)
        n62 = Select(t="UI: Front Panel State >> Close", s=w163, f="") -> (s? t:f=w166:string)
        n63 = call <vilib>:"Add State(s) to Queue__jki_lib_state_machine.vi"("State(s) in (\"\")"=w166, "State(s) at Back (\"\")"="Data: Cleanup\nExit") -> ("States Out"=w164:string)  [unwired: 13 in]
        n64 = call <vilib>:"Add State(s) to Queue__jki_lib_state_machine.vi"("State(s) in Front (\"\")"=w164, "State(s) in (\"\")"=w171) -> ("States Out"=w170:string)  [unwired: 13 in]
      }
      frame "---------- New Category ----------" {
        # "Template Separator\n(You can make a copy of, or modify, this frame)"
        n65 = call <vilib>:"Add State(s) to Queue__jki_lib_state_machine.vi"("State(s) in (\"\")"=w175) -> ("States Out"=w174:string)  [unwired: 14 in]
      }
    }
  }
